vi "Windmill_Hardware_acquiire_position.vi"(8 "error in (no error)":errorcluster, 11 "WindmillDevice in":refnum<class "WindmillDevice.lvclass">) -> (0 "error out":errorcluster, 3 "WindmillDevice out":refnum<class "WindmillDevice.lvclass">)   [LabVIEW 2020, in "WindmillDevice.lvclass"]
uses:
  WindmillDevice.lvclass
  C:/GEECS/Developers Version/source/Device Drivers/BaseDriver/BaseDriver.lvclass
  WindmillDevice.lvclass/WindmillDevice.ctl
  source/Device Drivers/BaseDriver/BaseDriver.lvclass
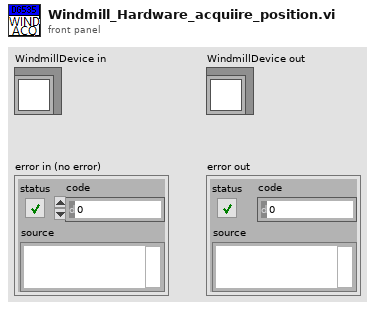
[diagram p1: front panel]
types:
  T1 = typedef "mysql_authentication.ctl" = cluster{"User":string, "Password":string, "Database":string}
  T2 = cluster{"Port":u16, "IP Address":string, "Authentication":T1}
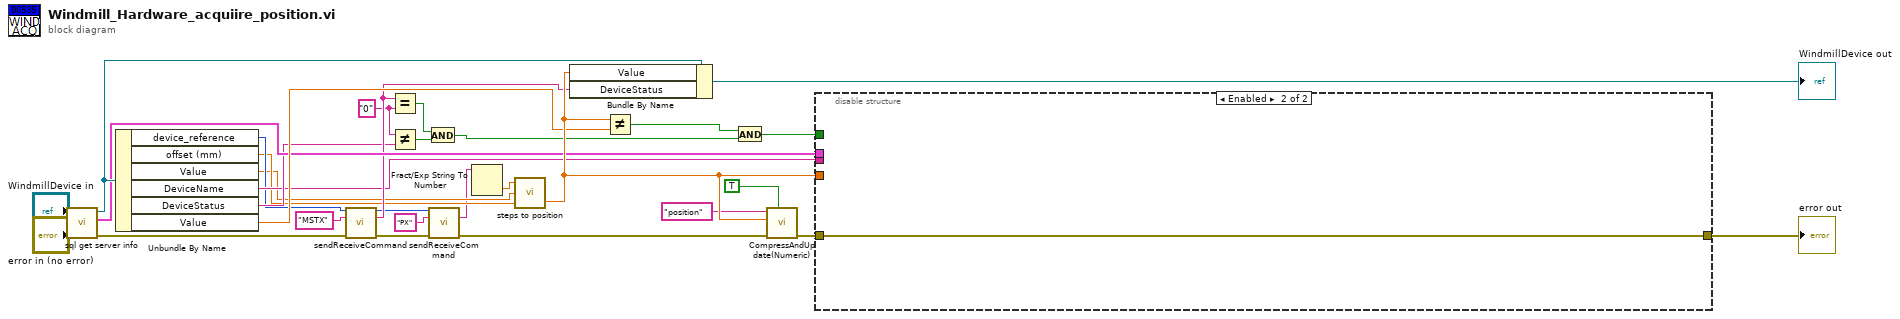
[diagram p0: block diagram]
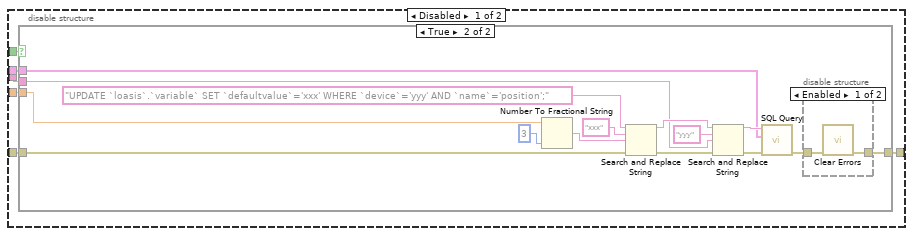
[diagram p2: hidden frame]
diagram:
  w16 = "0"
  n1 = call "sql get server info.vi"("error in (no error)"="error in (no error)", "BaseDriver in"="WindmillDevice in") -> ("error out"=w21:errorcluster, "SQL Server Info"=w20:T2, "BaseDriver out"=w29:refnum<class "WindmillDevice.lvclass">)  [unwired: 6 in, 1 out]
  n2 = Unbundle By Name ("pressure read")(w29) -> ("device_reference"=w11:i32, "offset (mm)"=w8:dbl, "Value"=w7:dbl, "DeviceName"=w13:string, "DeviceStatus"=w15:string, "Value"=w24:dbl)
  n3 = call "sendReceiveCommand.vi"("reference (in)"=w11, "write_string"="MSTX", "error in (no error)"=w21) -> ("reference (out)"=w12:i32, "read_string"=w19:string, "error out"=w10:errorcluster)  [unwired: 10 in]
  n4 = Equal?(x=w19, y=w16) -> (x = y?=w14:bool)
  n5 = Not Equal?(x=w16, y=w15) -> (x != y?=w17:bool)
  n6 = And(x=w14, y=w17) -> (x .and. y?=w23:bool)
  n7 = call "sendReceiveCommand.vi"("reference (in)"=w12, "write_string"="PX", "error in (no error)"=w10) -> ("read_string"=w2:string, "error out"=w4:errorcluster)  [unwired: 10 in, 1 out]
  n8 = Fract/Exp String To Number(string=w2) -> (number=w6:dbl)  [unwired: 3 in, 1 out]
  n9 = call "steps to position.vi"("Offset (mm)"=w8, "Pitch"=w7, "position (steps)"=w6) -> ("Position  (mm)"=w25:dbl)  [unwired: 1 in]
  n10 = Bundle By Name(cluster=w29, "Value"=w25, "DeviceStatus"=w19) -> (→"WindmillDevice out":refnum<class "WindmillDevice.lvclass">)
  n11 = Not Equal?(x=w25, y=w24) -> (x != y?=w26:bool)
  n12 = And(x=w26, y=w23) -> (x .and. y?=w27:bool)
  n13 = call "CompressAndUpdate(Numeric).vi"("force CVT update (false)"=TRUE, "error in"=w4, "Numeric"=w25, "command or variable name"="position") -> ("error out"=w18:errorcluster)  [unwired: 7 in]
  n14 = disable-structure shown="Enabled" {
    disable-tunnel: w13 -> [w37 _]
    disable-tunnel: w18 -> [w36 w57]
    disable-tunnel: w20 -> [w35 _]
    disable-tunnel: [w34 w57] -> w22
    disable-tunnel: w25 -> [w33 _]
    disable-tunnel: w27 -> [w32 _]
    frame Disabled {
      n15 = case shown="True" w32 {
        tunnel: [w38 w39] -> w34
        tunnel: w33 -> [_ w51]
        tunnel: w37 -> [_ w45]
        tunnel: w36 -> [w38 w44]
        tunnel: w35 -> [_ w41]
        frame False {
        }
        frame True {
          n16 = Number To Fractional String(number=w51, precision (6)=i16 3) -> (F-format string=w49:string)  [unwired: 2 in]
          n17 = Search and Replace String(input string="UPDATE `loasis`.`variable` SET `defaultvalue`='xxx' WHERE `device`='yyy' AND `name`='position';" ("Query"), search string="xxx", replace string=w49, error in=w44) -> (result string=w47:string, error out=w43:errorcluster)  [unwired: 4 in, 2 out]
          n18 = Search and Replace String(input string=w47, search string="yyy", replace string=w45, error in=w43) -> (result string=w46:string, error out=w42:errorcluster)  [unwired: 4 in, 2 out]
          n19 = call "SQL Query.vi"("error in (no error)"=w42, "SQL Server Info"=w41, "Query"=w46) -> ("error out"=w40:errorcluster)  [unwired: 7 in, 1 out]
          n20 = disable-structure shown="Enabled" {
            disable-tunnel: w40 -> [w55 w56]
            disable-tunnel: [w54 w56] -> w39
            frame Enabled {
              n21 = call "Clear Errors.vi"("error in (no error)"=w55) -> ("error out"=w54:errorcluster)  [unwired: 5 in, 1 out]
            }
            frame Disabled {
            }
          }
        }
      }
    }
    frame Enabled {
    }
  }
  "error out" <- w22
